vi "Set_Measurement_Time_Delay.vi"(7 "I2C Channel":u8, 8 "error in (no error)":errorcluster, 10 "Time Delay (ms)":u8=1 min=1 step=1, 11 "LINX Resource In":T1) -> (0 "error out":errorcluster, 3 "LINX Resource Out":T1)   [LabVIEW 2014, in "LMH-LINX.lvlib" / "HMC6352.lvlib"]
uses:
  <vilib>/MakerHub/LINX/Public/Sensors/Orientation/Compass/HMC6352/HMC6352.lvlib
  <vilib>/MakerHub/LINX/Private/Type Defs/LINX Ref.ctl
  <vilib>/MakerHub/LINX/Private/Type Defs/Platform.ctl
  <vilib>/MakerHub/LINX/Private/Type Defs/Interface.ctl
  <vilib>/MakerHub/LINX/Private/Device/Type Defs/LINX Device Config.ctl
  <vilib>/MakerHub/LINX/Private/Device/Type Defs/TCP Config.ctl
  <vilib>/MakerHub/LINX/Private/Device/Type Defs/Channels.ctl
  <vilib>/MakerHub/LINX/LMH-LINX.lvlib
  <vilib>/MakerHub/LINX/Private/Device/Device.lvlib
panel:
  # "INPUTS"
  # "OUTPUTS"
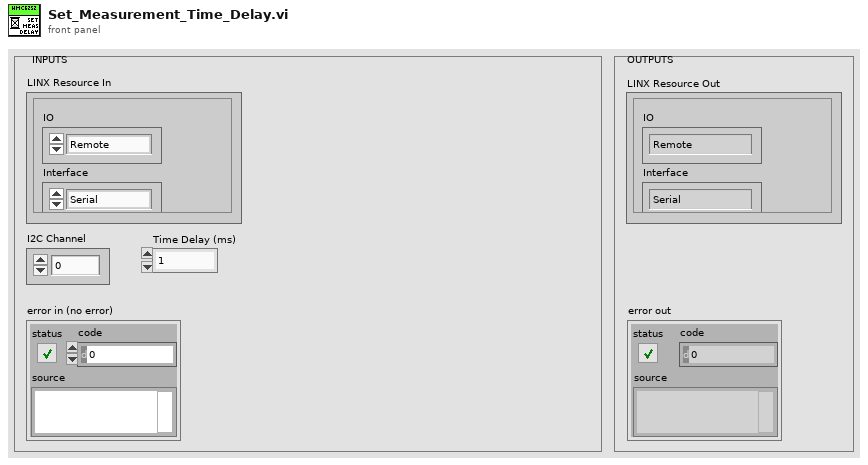
[diagram p1: front panel]
types:
  T1 = typedef "LMH-LINX.lvlib/LINX Ref.ctl" = cluster{"IO":T2, "Interface":T3, "LINX Device Config":T4}
  T2 = typedef "LMH-LINX.lvlib/Platform.ctl" = enum16{"Remote", "Local"}
  T3 = typedef "LMH-LINX.lvlib/Interface.ctl" = enum16{"Serial", "TCP"}
  T4 = typedef "LMH-LINX.lvlib/Device.lvlib/LINX Device Config.ctl" = cluster{"Interface":T3, "COM Port":refnum<visa-resource-name>, "TCP Configuration":T5, "Device Family":u8, "Device ID":u8, "Device Name":string, "TCP Ref":refnum<k5>, "Channels":T6}
  T5 = typedef "LMH-LINX.lvlib/Device.lvlib/TCP Config.ctl" = cluster{"IP Address":string, "Port":u16}
  T6 = typedef "LMH-LINX.lvlib/Channels.ctl" = cluster{"DI":u8[], "DO":u8[], "AI":u8[], "AO":u8[], "PWM":u8[], "QE":u8[], "UART":u8[], "I2C 2":u8[], "SPI":u8[], "CAN":u8[], "Servo":u8[], "AI Ref (V)":dbl, "AI Resolution (Bits)":u8, "AO Ref (V)":dbl, "AO Resolution (Bits)":u8}
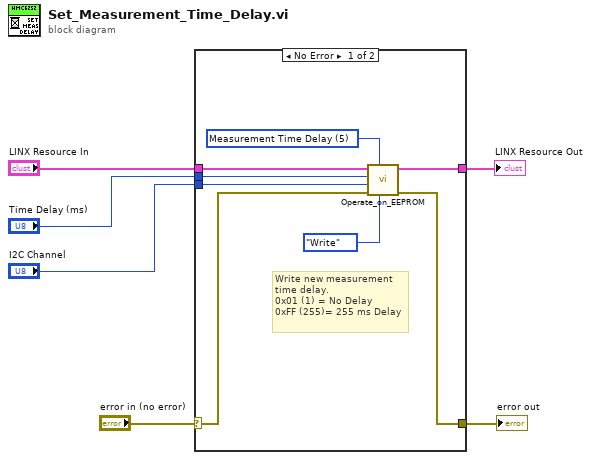
[diagram p0: block diagram]
diagram:
  n1 = case shown="No Error" "error in (no error)" {
    selector: "error in (no error)" -> [w12 w16]
    tunnel: [w7 w16] -> w5
    tunnel: "LINX Resource In" -> [w14 w15]
    tunnel: "Time Delay (ms)" -> [w10 _]
    tunnel: "I2C Channel" -> [w11 _]
    tunnel: [w8 w15] -> w1
    frame No Error {
      w9 = u8 5 items=["I2C Slave Address", "Magnetometer X Offset MSB", "Magnetometer X Offset LSB", "Magnetometer Y Offset MSB", "Magnetometer Y Offset LSB", "Measurement Time Delay", "Number of Summed Measurements", "Software Version Number", "Operation Mode Byte"] ("EEPROM Addresses")
      # "Write new measurement\ntime delay.\n0x01 (1) = No Delay\n0xFF (255)= 255 ms Delay"
      n2 = call <vilib>:"Operate_on_EEPROM.vi"("Operation"=enum16{"Write", "Read"}."Write", "EEPROM Addresses"=w9, "error in (no error)"=w12, "I2C Channel"=w11, "Data"=w10, "LINX Resource In"=w14) -> ("error out"=w7:errorcluster, "LINX Resource Out"=w8:T1)  [unwired: 3 in, 1 out]
    }
    frame Error {
    }
  }
  "error out" <- w5
  "LINX Resource Out" <- w1
